vi "Set IP Address.vi"(8 "error in (no error)":errorcluster, 9 "Reconnect Ethernet":bool, 10 "IP Address":string, 11 "ENET in":refnum<class "ENET_BS1200.lvclass">) -> (0 "error out":errorcluster, 3 "ENET out":refnum<class "ENET_BS1200.lvclass">)   [LabVIEW 2021, in "BS120x Driver.lvlib" / "ENET_BS1200.lvclass"]
uses:
  ENET_BS1200.lvclass
  ENET_BS1200.lvclass/ENET_BS1200.ctl
  <vilib>/nisyscfg/nisyscfg.lvlib
  <resource>/objmgr/nisysapi.rc
  <vilib>/nisyscfg/Save Changes (System).vi
  <vilib>/nisyscfg/Close (System).vi
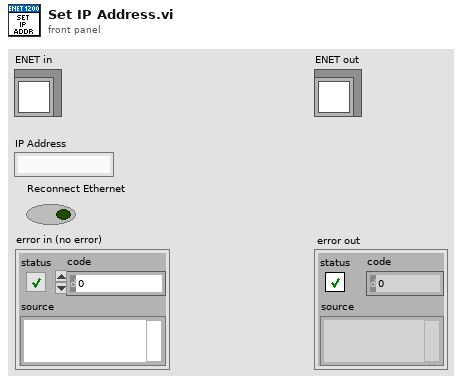
[diagram p1: front panel]
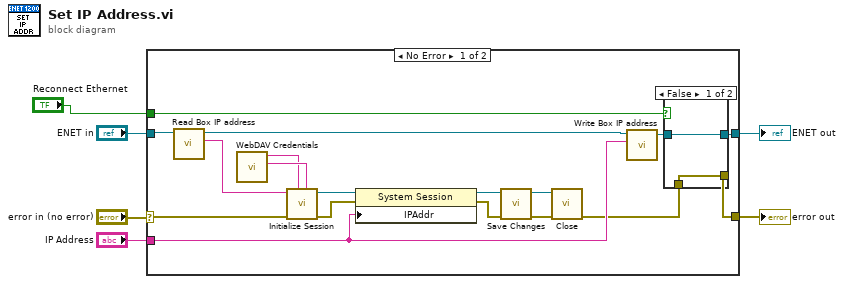
[diagram p0: block diagram]
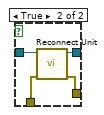
[diagram p2: hidden frame]
diagram:
  n1 = case shown="No Error" "error in (no error)" {
    selector: "error in (no error)" -> [w22 w32]
    tunnel: [w8 w32] -> w6
    tunnel: [w10 w31] -> w5
    tunnel: "ENET in" -> [w15 w31]
    tunnel: "IP Address" -> [w12 _]
    tunnel: "Reconnect Ethernet" -> [w7 _]
    frame No Error {
      n2 = call-dynamic "Read Box IP address.vi"("ENET_BS120x in"=w15) -> ("Box IP address"=w14:string, "ENET_BS120x out"=w13:refnum<class "ENET_BS1200.lvclass">)  [unwired: 8 in, 1 out]
      n3 = call "WebDAV Credentials.vi"() -> ("Password"=w24:string, "Username"=w23:string)  [unwired: 10 in]
      n4 = call <vilib>:"Initialize Session.vi"("Password"=w24, "User Name"=w23, "error in (no error)"=w22, "Target (localhost)"=w14) -> ("error out"=w21:errorcluster, "Session out"=w20:refnum<k21>)  [unwired: 6 in]
      n5 = property class="System Session"(reference=w20, error in=w21, "IPAddr"=w12) -> (reference out=w18:refnum<k21>, error out=w19:errorcluster)
      n6 = call-poly <vilib>:"Save Changes.vi"("error in (no error)"=w19, "Session in"=w18) -> ("error out"=w17:errorcluster, "Session out"=w16:refnum<k21>)  [unwired: 6 in, 2 out]
      n7 = call-poly <vilib>:"Close.vi"("error in (no error)"=w17, "Session in"=w16) -> ("error out"=w9:errorcluster)  [unwired: 9 in]
      n8 = call-dynamic "Write Box IP address.vi"("Box IP address"=w12, "ENET_BS120x in"=w13) -> ("ENET_BS120x out"=w11:refnum<class "ENET_BS1200.lvclass">)  [unwired: 8 in, 1 out]
      n9 = case shown="False" w7 {
        tunnel: w11 -> [w26 w30]
        tunnel: [w26 w29] -> w10
        tunnel: w9 -> [w25 w28]
        tunnel: [w25 w27] -> w8
        frame False {
        }
        frame True {
          n10 = call-dynamic "Reconnect Unit.vi"("error in (no error)"=w28, "ENET_BS120x in"=w30) -> ("error out"=w27:errorcluster, "ENET_BS120x out"=w29:refnum<class "ENET_BS1200.lvclass">)  [unwired: 8 in]
        }
      }
    }
    frame Error {
    }
  }
  "error out" <- w6
  "ENET out" <- w5
